vi "Teleop - Davis.vi"(10 "Match Info":T1={"Autonomous Elapsed Seconds"=0.0, "TeleOp Elapsed Seconds"=0.0, "Disabled Elapsed Seconds"=0.0, "Visited Autonomous"=FALSE, "Visited TeleOp"=FALSE, "Visited Disabled"=FALSE, "Autonomous Settings"={"Autonomous Style"=enum."Independent", "VI Refnum"=refnum}}, 11 "Call Context":T2) -> ()   [LabVIEW 2018]
doc: "This VI is called for each TeleOp packet received from the DS where the robot is not disabled. It is often used to read from the joysticks and update I/O or to update setpoints for timed control loops. It should complete and return within 20 milliseconds or it may miss DS packets."
uses:
  <vilib>/Rock Robotics/Network Tables/NT Write Numeric Array.vi
  <vilib>/Rock Robotics/Network Tables/NT Read Boolean.vi
  Robot Global Data.vi
  <vilib>/Rock Robotics/WPI/ThirdParty/Phoenix-LabVIEW/Motor Controller/Controls/CTRE_Phoenix_MotorControl_ControlMode.ctl
  <vilib>/Rock Robotics/WPI/Solenoid/WPI_SolenoidSetEnum.vi
  <vilib>/Rock Robotics/WPI/Solenoid/WPI_SolenoidValue.ctl
  <vilib>/Rock Robotics/Network Tables/NT Write Boolean.vi
  <vilib>/Rock Robotics/Network Tables/NT Write Number.vi
  <vilib>/Rock Robotics/WPI/ThirdParty/Phoenix-LabVIEW/Motor Controller/Get/CTRE_Phoenix_MotorController_GetSelectedSensorData.vi
  <vilib>/functionblocks/FB Core/FB Core.xnode
  <vilib>/functionblocks/Bistables/SR Bistable/SR Bistable.vi
  <vilib>/functionblocks/NI_FunctionBlock Libraries.lvlib
  <vilib>/Rock Robotics/Network Tables/NT Read Number.vi
  <vilib>/Rock Robotics/Network Tables/NT Write Boolean Array.vi
  <vilib>/Rock Robotics/WPI/DriverStation/WPI_DriverStationMatch Info.ctl
  <vilib>/Rock Robotics/WPI/DriverStation/WPI_DriverStationDerivedRobotMode.ctl
panel:
  in  "I Zone":dbl
  in  "F - Generally is zero for position-servo":dbl
  in  "D":dbl
  in  "I":dbl
  in  "P":dbl
  out "Sample Slider 0":dbl(slide) scale=0.0..5.0
  out "Sample Boolean 1":bool
  out "Sample Boolean 0":bool
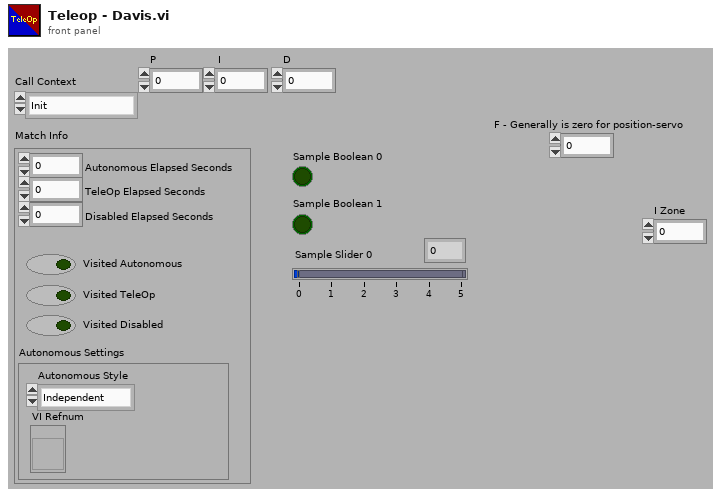
[diagram p1: front panel]
types:
  T1 = typedef "WPI_DriverStationMatch Info.ctl" = cluster{"Autonomous Elapsed Seconds":dbl, "TeleOp Elapsed Seconds":dbl, "Disabled Elapsed Seconds":dbl, "Visited Autonomous":bool, "Visited TeleOp":bool, "Visited Disabled":bool, "Autonomous Settings":cluster{"Autonomous Style":enum16{"Iterative", "Independent"}, "VI Refnum":refnum<vi>}}
  T2 = typedef "WPI_DriverStationDerivedRobotMode.ctl" = enum16{"Init", "Execute", "Stop"}
  T3 = typedef "CTRE_Phoenix_MotorControl_ControlMode.ctl" = u16
  T4 = typedef "WPI_MotorControlDeviceRef.ctl" = cluster{"DeviceStatus":errorcluster, "Type":T5, "PWM":cluster{"PWM Channel":T6, "DeadBand":T7}, "CAN":cluster{"Device Number":u8, "SetOutput VI Ref":variant, "GetOutput VI Ref":variant, "Enable VI Ref":variant, "Disable VI Ref":variant, "Data":variant}, "Invert":bool, "DIO PWM":cluster{"PWM \"Enable\" Channel":T6, "DIOChannel":T8, "PWM Rate":dbl}}
  T5 = typedef "WPI_MotorControlType.ctl" = enum16{"PWM", "CAN", "DIO PWM"}
  T6 = typedef "FPGA_DIOPWMChannel.ctl" = enum8{"PWM 0", "PWM 1", "PWM 2", "PWM 3", "PWM 4", "PWM 5", "PWM 6", "PWM 7", "PWM 8", "PWM 9", "PWM MXP 0", "PWM MXP 1", "PWM MXP 2", "PWM MXP 3", "PWM MXP 4", "PWM MXP 5", "PWM MXP 6", "PWM MXP 7", "PWM MXP 8", "PWM MXP 9", "Invalid"}
  T7 = typedef "WPI_PWMDeadband.ctl" = cluster{"Name":string, "maxPositivePwm":i32, "minPositivePwm":i32, "centerPwm":i32, "maxNegativePwm":i32, "minNegativePwm":i32, "angularRange":u16}
  T8 = typedef "FPGA_DIOChannel.ctl" = enum8{"DIO 0", "DIO 1", "DIO 2", "DIO 3", "DIO 4", "DIO 5", "DIO 6", "DIO 7", "DIO 8", "DIO 9", "DIO MXP 0", "DIO MXP 1", "DIO MXP 2", "DIO MXP 3", "DIO MXP 4", "DIO MXP 5", "DIO MXP 6", "DIO MXP 7", "DIO MXP 8", "DIO MXP 9", "DIO MXP 10", "DIO MXP 11", "DIO MXP 12", "DIO MXP 13", "DIO MXP 14", "DIO MXP 15", "SPI Port CS1", "SPI Port CS2", "SPI Port CS3", "SPI Port MISO", "SPI Port MOSI", "Invalid"}
  T9 = typedef "WPI_SwitchDevRef.ctl" = cluster{"DevStatus":errorcluster, "DIO Channel":T8, "CntIndex":T10, "Normally Closed":bool}
  T10 = typedef "FPGA_CounterCtrSystemIndex.ctl" = enum8{"Ctr 0", "Ctr 1", "Ctr 2", "Ctr 3", "Ctr 4", "Ctr 5", "Ctr 6", "Ctr 7", "Invalid"}
  T11 = typedef "WPI_SolenoidValue.ctl" = enum16{"Off", "On", "Forward", "Reverse"}
  T12 = typedef "WPI_SolenoidDevRef.ctl" = cluster{"DevStatus":errorcluster, "Pneumatics Control Module":u8, "Forward Solenoid Channel":T13, "Reverse Solenoid Channel":T13}
  T13 = typedef "WPI_SolenoidChannel.ctl" = enum8{"Solenoid 0", "Solenoid 1", "Solenoid 2", "Solenoid 3", "Solenoid 4", "Solenoid 5", "Solenoid 6", "Solenoid 7", "Invalid"}
  T14 = typedef "WPI_JoystickDevRef.ctl" = cluster{"Device":T15}
  T15 = typedef "WPI_JoystickDeviceEnum.ctl" = enum16{"USB 0", "USB 1", "USB 2", "USB 3", "USB 4", "USB 5"}
  T16 = typedef "WPI_RobotDriveDevRef.ctl" = cluster{"DevStatus":errorcluster, "Motors[]":T4[], "Square Inputs":bool, "Max Output":dbl}
  T17 = cluster{"JoystickDevRef":T14, "JoystickDevRef":T14}
  T18 = cluster{"Axes[0]":dbl, "Axes[1]":dbl, "Axes[2]":dbl, "Axes[3]":dbl, "Axes[4]":dbl, "Axes[5]":dbl, "Axes[6]":dbl, "Axes[7]":dbl, "Axes[8]":dbl}
  T19 = cluster{"Buttons[0]":bool, "Buttons[1]":bool, "Buttons[2]":bool, "Buttons[3]":bool, "Buttons[4]":bool, "Buttons[5]":bool, "Buttons[6]":bool, "Buttons[7]":bool, "Buttons[8]":bool}
  T20 = typedef "WPI_ServoDeviceRef.ctl" = cluster{"DeviceStatus":errorcluster, "PWM Channel":T6, "DeadBand":T7}
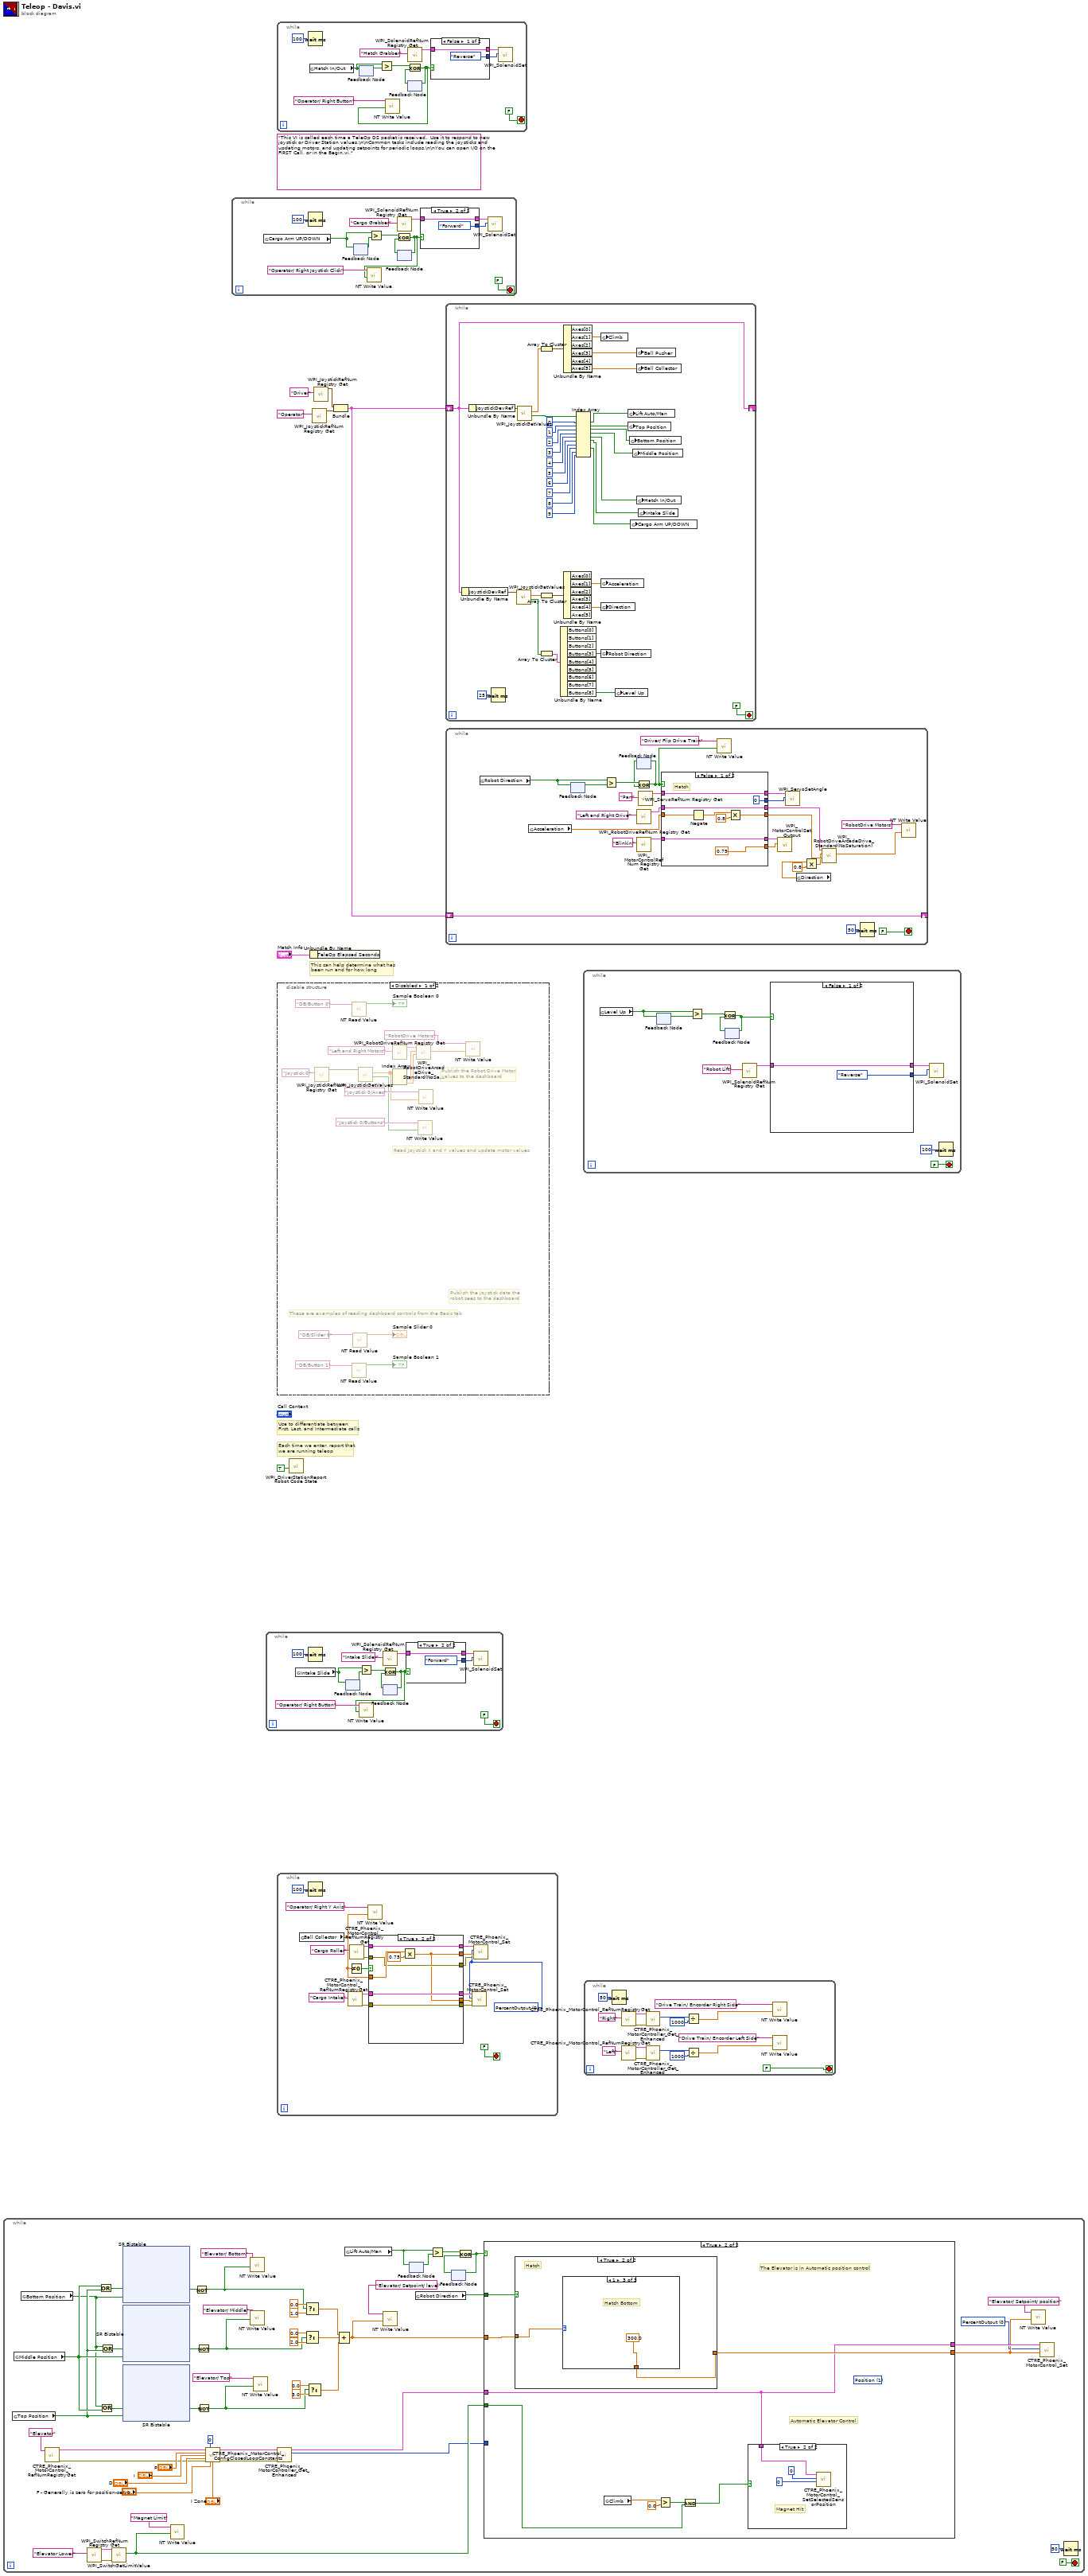
[diagram p0: block diagram]
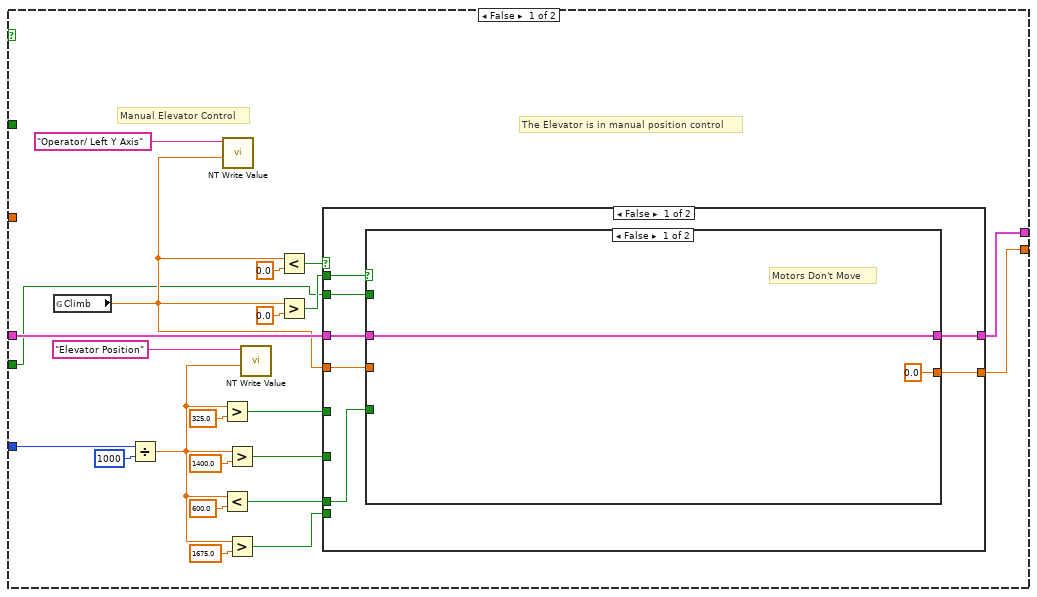
[diagram p2: hidden frame]
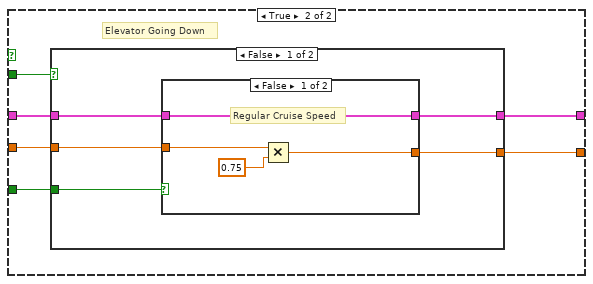
[diagram p3: hidden frame]
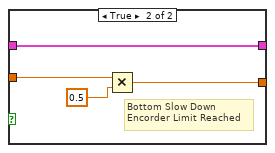
[diagram p4: hidden frame]
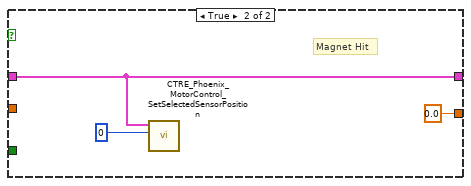
[diagram p5: hidden frame]
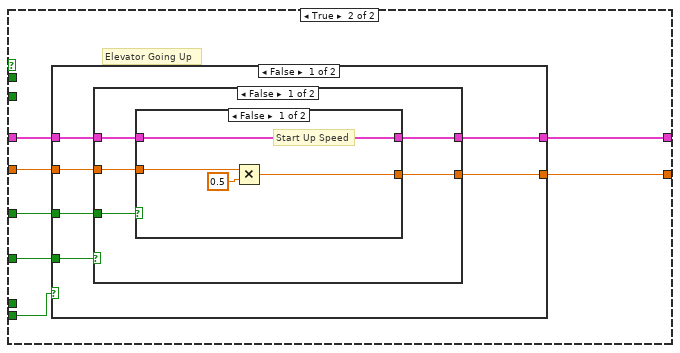
[diagram p6: hidden frame]
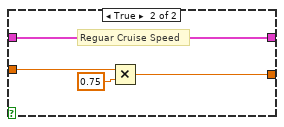
[diagram p7: hidden frame]
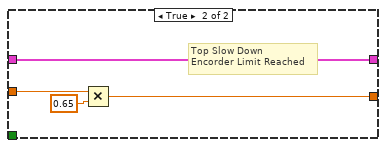
[diagram p8: hidden frame]
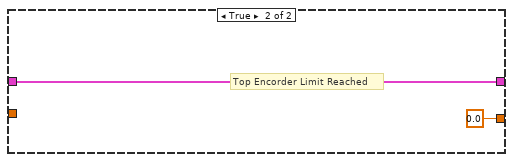
[diagram p9: hidden frame]
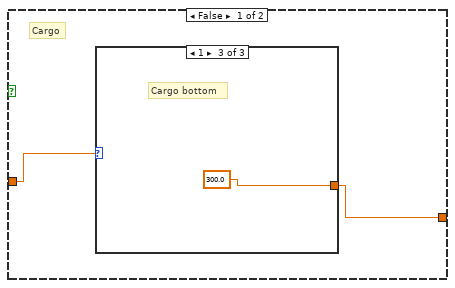
[diagram p11: hidden frame]
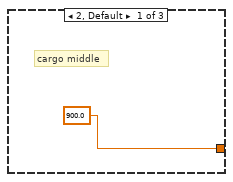
[diagram p12: hidden frame]
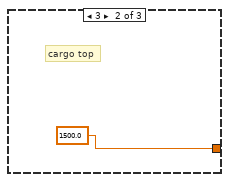
[diagram p13: hidden frame]
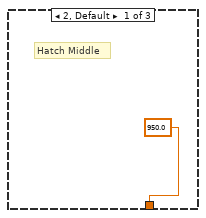
[diagram p14: hidden frame]
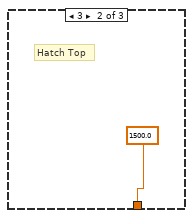
[diagram p15: hidden frame]
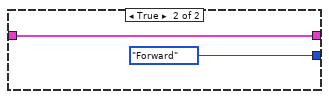
[diagram p16: hidden frame]
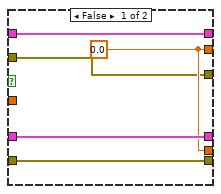
[diagram p17: hidden frame]
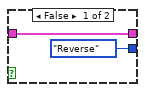
[diagram p18: hidden frame]
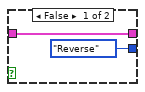
[diagram p19: hidden frame]
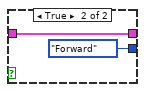
[diagram p20: hidden frame]
diagram:
  (unwired) "This VI is called each time a TeleOp DS packet is received.  Use it to respond to new joystick or Driver Station values.\n\nCommon tasks include reading the joysticks and updating motors, and updating setpoints for periodic loops.\n\nYou can open I/O on the FIRST Call, or in the Begin.vi."
  # "Each time we enter, report that\nwe are running teleop"
  # "Use to differentiate between\nFirst, Last, and Intermediate calls"
  # "This can help determine what has\nbeen run and for how long"
  n1 = while {
    stop <- FALSE stop-if-true
    w8 = T3 0 items=["PercentOutput"=0, "Position"=1, "Velocity"=2, "Current"=3, "Follower"=5, "MotionProfile"=6, "MotionMagic"=7, "MotionProfileArc"=10, "Disabled"=15] ("Control Mode")
    n2 = global read "Robot Global Data.vi" "Top Position"() -> (w12:bool)
    n3 = global read "Robot Global Data.vi" "Middle Position"() -> (w13:bool)
    n4 = global read "Robot Global Data.vi" "Bottom Position"() -> (w11:bool)
    n5 = call <vilib>:"CTRE_Phoenix_MotorControl_RefNumRegistryGet.vi"("refnum name"="Elevator") -> ("error out"=w20:errorcluster, "PhoenixMotorControlDevRef"=w31:T4)  [unwired: 9 in]
    n6 = call <vilib>:"WPI_SwitchRefNum Registry Get.vi"("refnum name"="Elevator Lower") -> ("error out"=w38:errorcluster, "SwitchDevRef"=w37:T9)  [unwired: 9 in]
    n7 = Or(x=w13, y=w12) -> (x .or. y?=w41:bool)
    n8 = Or(x=w11, y=w13) -> (x .or. y?=w39:bool)
    n9 = Or(x=w11, y=w12) -> (x .or. y?=w40:bool)
    n10 = call <vilib>:"WPI_SwitchGetLimitValue.vi"("error in (no error)"=w38, "SwitchDevRef"=w37) -> ("Switch Pressed"=w34:bool)  [unwired: 7 in, 2 out]
    n11 = xnode "SR Bistable"("reset"=w41, "set"=w11) -> ("output"=w18:bool)  [unwired: 1 in, 1 out]
    n12 = xnode "SR Bistable"("reset"=w40, "set"=w13) -> ("output"=w17:bool)  [unwired: 1 in, 1 out]
    n13 = xnode "SR Bistable"("reset"=w39, "set"=w12) -> ("output"=w16:bool)  [unwired: 1 in, 1 out]
    n14 = call-poly <vilib>:"NT Write Value.vi"("Boolean"=w34, "Name"="Magnet Limit") -> ()  [unwired: 9 in, 1 out]
    n15 = Not(x=w18) -> (.not. x?=w10:bool)
    n16 = Not(x=w17) -> (.not. x?=w14:bool)
    n17 = Not(x=w16) -> (.not. x?=w15:bool)
    n18 = call <vilib>:"CTRE_Phoenix_MotorControl_ConfigClosedLoopConstants.vi"("PhoenixMotorControlDevRef"=w31, "slotIdx"=0, "P"="P", "I"="I", "D"="D", "error in (no error)"=w20, "F"="F - Generally is zero for position-servo", "I Zone"="I Zone") -> ("PhoenixMotorControlDevRef"=w32:T4, "error out"=w19:errorcluster)  [unwired: 6 in]
    n19 = call-poly <vilib>:"NT Write Value.vi"("Boolean"=w14, "Name"="Elevator/ Middle") -> ()  [unwired: 9 in, 1 out]
    n20 = call-poly <vilib>:"NT Write Value.vi"("Boolean"=w10, "Name"="Elevator/ Bottom") -> ()  [unwired: 9 in, 1 out]
    n21 = call-poly <vilib>:"NT Write Value.vi"("Boolean"=w15, "Name"="Elevator/ Top") -> ()  [unwired: 9 in, 1 out]
    n22 = call-poly <vilib>:"CTRE_Phoenix_MotorController_Get_Enhanced.vi"("PhoenixMotorControlDevRef"=w32, "error in"=w19) -> ("PhoenixMotorControlDevRef"=w9:T4, "Position (Raw Sensor Units)"=w33:i32)  [unwired: 10 in, 2 out]
    n23 = Select(t=0.0, s=w10, f=1.0) -> (s? t:f=w53:dbl)
    n24 = Select(t=0.0, s=w14, f=2.0) -> (s? t:f=w52:dbl)
    n25 = Select(t=0.0, s=w15, f=3.0) -> (s? t:f=w51:dbl)
    n26 = Compound Arithmetic op=ADD(w53, w52, w51) -> (w23:dbl)
    n27 = global read "Robot Global Data.vi" "Lift Auto/Man"() -> (w55:bool)
    n28 = call-poly <vilib>:"NT Write Value.vi"("Numeric"=w23, "Name"="Elevator/ Setpoint/ level") -> ()  [unwired: 9 in, 1 out]
    n29 = feedback #1() -> (w57:bool)  [unwired: 1 in]
    n30 = feedback-in #1(w55) -> ()
    n31 = global read "Robot Global Data.vi" "Robot Direction"() -> (w54:bool)
    n32 = Greater?(x=w55, y=w57) -> (0:w58:bool)
    n33 = feedback #2() -> (w59:bool)  [unwired: 1 in]
    n34 = Exclusive Or(1:w59, 2:w58) -> (0:w56:bool)
    n35 = feedback-in #2(w56) -> ()
    n36 = case shown="True" w56 {
      tunnel: [w206 w276] -> w21
      tunnel: w9 -> [w205 w275]
      tunnel: [w204 w275] -> w60
      tunnel: w33 -> [w190 _]
      tunnel: w54 -> [_ w283]
      tunnel: w23 -> [_ w282]
      tunnel: w34 -> [w191 w279]
      frame False {
        # "The Elevator is in manual position control"
        # "Manual Elevator Control"
        n37 = global read "Robot Global Data.vi" "Climb"() -> (w197:dbl)
        n38 = Divide(x=w190, y=1000) -> (x/y=w196:dbl)
        n39 = Greater?(x=w196, y=325.0) -> (0:w194:bool)
        n40 = Less?(x=w196, y=600.0) -> (x < y?=w192:bool)
        n41 = call-poly <vilib>:"NT Write Value.vi"("Numeric"=w197, "Name"="Operator/ Left Y Axis") -> ()  [unwired: 9 in, 1 out]
        n42 = Greater?(x=w196, y=1400.0) -> (0:w198:bool)
        n43 = Greater?(x=w196, y=1675.0) -> (0:w199:bool)
        n44 = call-poly <vilib>:"NT Write Value.vi"("Numeric"=w196, "Name"="Elevator Position") -> ()  [unwired: 9 in, 1 out]
        n45 = Less?(x=w197, y=0.0) -> (x < y?=w200:bool)
        n46 = Greater?(x=w197, y=0.0) -> (0:w193:bool)
        n47 = case shown="False" w200 {
          tunnel: [w216 w246] -> w206
          tunnel: w205 -> [w214 w247]
          tunnel: [w215 w248] -> w204
          tunnel: w199 -> [_ w249]
          tunnel: w198 -> [_ w245]
          tunnel: w197 -> [w212 w244]
          tunnel: w194 -> [_ w243]
          tunnel: w193 -> [w218 _]
          tunnel: w191 -> [w217 _]
          tunnel: w192 -> [w213 _]
          frame False {
            n48 = case shown="False" w218 {
              tunnel: w217 -> [_ w226]
              tunnel: [0.0 ("Climb") w225] -> w216
              tunnel: [w220 w224] -> w215
              tunnel: w214 -> [w220 w223]
              tunnel: w213 -> [_ w222]
              tunnel: w212 -> [_ w221]
              frame False {
                # "Motors Don't Move"
              }
              frame True {
                # "Elevator Going Down"
                n49 = case shown="False" w226 {
                  tunnel: [w230 0.0 ("Climb")] -> w225
                  tunnel: [w228 w240] -> w224
                  tunnel: w223 -> [w227 w240]
                  tunnel: w222 -> [w231 _]
                  tunnel: w221 -> [w229 _]
                  frame False {
                    n50 = case shown="False" w231 {
                      tunnel: [w235 w239] -> w230
                      tunnel: w229 -> [w234 w238]
                      tunnel: [w233 w236] -> w228
                      tunnel: w227 -> [w233 w236]
                      frame False {
                        # "Regular Cruise Speed"
                        n51 = Multiply(x=w234, y=0.75) -> (x*y=w235:dbl)
                      }
                      frame True {
                        # "Bottom Slow Down\nEncorder Limit Reached"
                        n52 = Multiply(x=w238, y=0.5) -> (x*y=w239:dbl)
                      }
                    }
                  }
                  frame True {
                    # "Magnet Hit"
                    n53 = call <vilib>:"CTRE_Phoenix_MotorControl_SetSelectedSensorPosition.vi"("New Sensor Position"=0, "PhoenixMotorControlDevRef"=w240) -> ()  [unwired: 8 in, 2 out]
                  }
                }
              }
            }
          }
          frame True {
            # "Elevator Going Up"
            n54 = case shown="False" w249 {
              tunnel: [w254 w274] -> w248
              tunnel: w247 -> [w253 w274]
              tunnel: [w252 0.0 ("Climb")] -> w246
              tunnel: w245 -> [w255 _]
              tunnel: w244 -> [w251 _]
              tunnel: w243 -> [w250 _]
              frame False {
                n55 = case shown="False" w255 {
                  tunnel: [w257 w272] -> w254
                  tunnel: w253 -> [w256 w272]
                  tunnel: [w259 w271] -> w252
                  tunnel: w251 -> [w258 w270]
                  tunnel: w250 -> [w260 _]
                  frame False {
                    n56 = case shown="False" w260 {
                      tunnel: [w264 w268] -> w259
                      tunnel: w258 -> [w263 w267]
                      tunnel: [w261 w266] -> w257
                      tunnel: w256 -> [w261 w266]
                      frame False {
                        # "Start Up Speed"
                        n57 = Multiply(x=w263, y=0.5) -> (x*y=w264:dbl)
                      }
                      frame True {
                        # "Reguar Cruise Speed"
                        n58 = Multiply(x=w267, y=0.75) -> (x*y=w268:dbl)
                      }
                    }
                  }
                  frame True {
                    # "Top Slow Down\nEncorder Limit Reached"
                    n59 = Multiply(x=w270, y=0.65) -> (x*y=w271:dbl)
                  }
                }
              }
              frame True {
                # "Top Encorder Limit Reached"
              }
            }
          }
        }
      }
      frame True {
        (unwired) T3 1 items=["PercentOutput"=0, "Position"=1, "Velocity"=2, "Current"=3, "Follower"=5, "MotionProfile"=6, "MotionMagic"=7, "MotionProfileArc"=10, "Disabled"=15] ("Control Mode")
        # "The Elevator is in Automatic position control"
        # "Automatic Elevator Control"
        n60 = case shown="True" w283 {
          tunnel: w282 -> [w288 w293]
          tunnel: [w287 w292] -> w276
          frame False {
            # "Cargo"
            n61 = case shown="1" w288 {
              tunnel: [900.0 ("setpoint") 1500.0 ("setpoint") 300.0 ("setpoint")] -> w287
              frame 2, Default {
                # "cargo middle"
              }
              frame 3 {
                # "cargo top"
              }
              frame 1 {
                # "Cargo bottom"
              }
            }
          }
          frame True {
            # "Hatch"
            n62 = case shown="1" w293 {
              tunnel: [950.0 ("setpoint") 1500.0 ("setpoint") 300.0 ("setpoint")] -> w292
              frame 2, Default {
                # "Hatch Middle"
              }
              frame 3 {
                # "Hatch Top"
              }
              frame 1 {
                # "Hatch Bottom"
              }
            }
          }
        }
        n63 = global read "Robot Global Data.vi" "Climb"() -> (w280:dbl)
        n64 = Greater?(x=w280, y=0.0) -> (0:w278:bool)
        n65 = And(x=w278, y=w279) -> (x .and. y?=w277:bool)
        n66 = case shown="True" w277 {
          tunnel: w275 -> [_ w286]
          frame False {
          }
          frame True {
            # "Magnet Hit"
            n67 = call <vilib>:"CTRE_Phoenix_MotorControl_SetSelectedSensorPosition.vi"("pidLoopIdx"=u32 0, "New Sensor Position"=0, "PhoenixMotorControlDevRef"=w286) -> ()  [unwired: 7 in, 2 out]
          }
        }
      }
    }
    n68 = call-poly <vilib>:"NT Write Value.vi"("Numeric"=w21, "Name"="Elevator/ Setpoint/ position") -> ()  [unwired: 9 in, 1 out]
    n69 = call <vilib>:"CTRE_Phoenix_MotorControl_Set.vi"("Output"=w21, "Control Mode"=w8, "PhoenixMotorControlDevRef"=w60) -> ()  [unwired: 7 in, 2 out]
    n70 = Wait (ms)(milliseconds to wait=u32 50) -> ()  [unwired: 1 out]
  }
  n71 = while {
    stop <- FALSE stop-if-true
    n72 = global read "Robot Global Data.vi" "Cargo Arm UP/DOWN"() -> (w298:bool)
    n73 = Wait (ms)(milliseconds to wait=u32 100) -> ()  [unwired: 1 out]
    n74 = feedback #3() -> (w302:bool)  [unwired: 1 in]
    n75 = feedback-in #3(w298) -> ()
    n76 = Greater?(x=w298, y=w302) -> (0:w303:bool)
    n77 = call <vilib>:"WPI_SolenoidRefNum Registry Get.vi"("refnum name"="Cargo Grabber") -> ("SolenoidDevRef"=w306:T12)  [unwired: 9 in, 1 out]
    n78 = feedback #4() -> (w304:bool)  [unwired: 1 in]
    n79 = Exclusive Or(1:w304, 2:w303) -> (0:w297:bool)
    n80 = call-poly <vilib>:"NT Write Value.vi"("Boolean"=w297, "Name"="Operator/ Right Joystick Click") -> ()  [unwired: 9 in, 1 out]
    n81 = feedback-in #4(w297) -> ()
    n82 = case shown="True" w297 {
      tunnel: w306 -> [w310 w312]
      tunnel: [w310 w312] -> w307
      tunnel: [WPI_SolenoidValue."Reverse" ("Value") WPI_SolenoidValue."Forward" ("Value")] -> w308
      frame False {
      }
      frame True {
      }
    }
    n83 = call-poly <vilib>:"WPI_SolenoidSet.vi"("Value"=w308, "SolenoidDevRef"=w307) -> ()  [unwired: 8 in, 2 out]
  }
  n84 = while {
    stop <- FALSE stop-if-true
    n85 = global read "Robot Global Data.vi" "Intake Slide"() -> (w317:bool)
    n86 = Wait (ms)(milliseconds to wait=u32 100) -> ()  [unwired: 1 out]
    n87 = feedback #5() -> (w324:bool)  [unwired: 1 in]
    n88 = feedback-in #5(w317) -> ()
    n89 = Greater?(x=w317, y=w324) -> (0:w323:bool)
    n90 = call <vilib>:"WPI_SolenoidRefNum Registry Get.vi"("refnum name"="Intake Slider") -> ("SolenoidDevRef"=w320:T12)  [unwired: 9 in, 1 out]
    n91 = feedback #6() -> (w322:bool)  [unwired: 1 in]
    n92 = Exclusive Or(1:w322, 2:w323) -> (0:w313:bool)
    n93 = call-poly <vilib>:"NT Write Value.vi"("Boolean"=w313, "Name"="Operator/ Right Button") -> ()  [unwired: 9 in, 1 out]
    n94 = feedback-in #6(w313) -> ()
    n95 = case shown="True" w313 {
      tunnel: w320 -> [w326 w328]
      tunnel: [w326 w328] -> w319
      tunnel: [WPI_SolenoidValue."Reverse" ("Value") WPI_SolenoidValue."Forward" ("Value")] -> w318
      frame False {
      }
      frame True {
      }
    }
    n96 = call-poly <vilib>:"WPI_SolenoidSet.vi"("Value"=w318, "SolenoidDevRef"=w319) -> ()  [unwired: 8 in, 2 out]
  }
  n97 = while {
    stop <- FALSE stop-if-true
    n98 = Wait (ms)(milliseconds to wait=u32 100) -> ()  [unwired: 1 out]
    n99 = global read "Robot Global Data.vi" "Hatch In/Out"() -> (w330:bool)
    n100 = feedback #7() -> (w333:bool)  [unwired: 1 in]
    n101 = feedback-in #7(w330) -> ()
    n102 = Greater?(x=w330, y=w333) -> (0:w332:bool)
    n103 = call <vilib>:"WPI_SolenoidRefNum Registry Get.vi"("refnum name"="Hatch Grabber") -> ("SolenoidDevRef"=w339:T12)  [unwired: 9 in, 1 out]
    n104 = feedback #8() -> (w331:bool)  [unwired: 1 in]
    n105 = Exclusive Or(1:w331, 2:w332) -> (0:w329:bool)
    n106 = call-poly <vilib>:"NT Write Value.vi"("Boolean"=w329, "Name"="Operator/ Right Button") -> ()  [unwired: 9 in, 1 out]
    n107 = feedback-in #8(w329) -> ()
    n108 = case shown="False" w329 {
      tunnel: w339 -> [w342 w344]
      tunnel: [w342 w344] -> w338
      tunnel: [WPI_SolenoidValue."Reverse" ("Value") WPI_SolenoidValue."Forward" ("Value")] -> w337
      frame False {
      }
      frame True {
      }
    }
    n109 = call-poly <vilib>:"WPI_SolenoidSet.vi"("Value"=w337, "SolenoidDevRef"=w338) -> ()  [unwired: 8 in, 2 out]
  }
  n110 = disable-structure shown="Disabled" {
    frame Disabled {
      # "These are examples of reading dashboard controls from the Basic tab"
      # "Publish the Robot Drive Motor\nvalues to the dashboard"
      # "Publish the joystick data the\nrobot sees to the dashboard"
      # "Read Joystick X and Y values and update motor values"
      n111 = call <vilib>:"WPI_JoystickRefNum Registry Get.vi"("refnum name"="Joystick 0") -> ("JoystickDevRef"=w358:T14)  [unwired: 1 in, 9 out]
      n112 = call-poly <vilib>:"NT Read Value.vi"("Name"="DB/Button 0" ("refnum name")) -> ("Boolean"=→"Sample Boolean 0":bool)  [unwired: 9 in, 1 out]
      n113 = call-poly <vilib>:"NT Read Value.vi"("Name"="DB/Button 1" ("refnum name")) -> ("Boolean"=→"Sample Boolean 1":bool)  [unwired: 9 in, 1 out]
      n114 = call-poly <vilib>:"NT Read Value.vi"("Name"="DB/Slider 0" ("refnum name")) -> ("Numeric"=→"Sample Slider 0":dbl)  [unwired: 9 in, 1 out]
      n115 = call <vilib>:"WPI_JoystickGetValues.vi"("JoystickDevRef"=w358) -> ("Buttons"=w353:bool[], "Axes"=w354:dbl[])  [unwired: 6 in, 3 out]
      n116 = call <vilib>:"WPI_RobotDriveRefNum Registry Get.vi"("refnum name"="Left and Right Motors") -> ("RobotDriveDevRef"=w361:T16)  [unwired: 1 in, 9 out]
      n117 = Index Array(array=w354) -> (element #1=w360:dbl, element #2=w357:dbl)  [unwired: 2 in]
      n118 = call <vilib>:"WPI_RobotDriveArcadeDrive_Standard(NoSaturation).vi"("Y axis value"=w357, "X axis value"=w360, "RobotDriveDevRef"=w361) -> ("Motor Values"=w346:dbl[])  [unwired: 1 in, 7 out]
      n119 = call-poly <vilib>:"NT Write Value.vi"("Boolean Array"=w353, "Name"="Joystick 0/Buttons") -> ()  [unwired: 9 in, 1 out]
      n120 = call-poly <vilib>:"NT Write Value.vi"("Numeric Array"=w354, "Name"="Joystick 0/Axes") -> ()  [unwired: 9 in, 1 out]
      n121 = call-poly <vilib>:"NT Write Value.vi"("Numeric Array"=w346, "Name"="RobotDrive Motors") -> ()  [unwired: 9 in, 1 out]
    }
    frame Enabled {
    }
  }
  n122 = while {
    stop <- FALSE stop-if-true
    w368 = T3 0 items=["PercentOutput"=0, "Position"=1, "Velocity"=2, "Current"=3, "Follower"=5, "MotionProfile"=6, "MotionMagic"=7, "MotionProfileArc"=10, "Disabled"=15] ("Control Mode")
    n123 = global read "Robot Global Data.vi" "Ball Collector"() -> (w373:dbl)
    n124 = Wait (ms)(milliseconds to wait=u32 100) -> ()  [unwired: 1 out]
    n125 = call <vilib>:"CTRE_Phoenix_MotorControl_RefNumRegistryGet.vi"("refnum name"="Cargo Intake") -> ("error out"=w364:errorcluster, "PhoenixMotorControlDevRef"=w369:T4)  [unwired: 9 in]
    n126 = Not Equal To 0?(x=w373) -> (x != 0?=w380:bool)
    n127 = call <vilib>:"CTRE_Phoenix_MotorControl_RefNumRegistryGet.vi"("refnum name"="Cargo Roller") -> ("error out"=w366:errorcluster, "PhoenixMotorControlDevRef"=w377:T4)  [unwired: 9 in]
    n128 = call-poly <vilib>:"NT Write Value.vi"("Numeric"=w373, "Name"="Operator/ Right Y Axis") -> ()  [unwired: 9 in, 1 out]
    n129 = case shown="True" w380 {
      tunnel: w377 -> [w385 w392]
      tunnel: [w385 w392] -> w378
      tunnel: w373 -> [_ w391]
      tunnel: [w383 w386] -> w379
      tunnel: [w384 w389] -> w370
      tunnel: w369 -> [w384 w389]
      tunnel: [w381 w388] -> w367
      tunnel: w366 -> [w381 w388]
      tunnel: [w382 w387] -> w365
      tunnel: w364 -> [w382 w387]
      tunnel: [w383 w386] -> w363
      frame False {
        w383 = 0.0 ("Climb")
      }
      frame True {
        n130 = Multiply(x=w391, y=0.75) -> (x*y=w386:dbl)
      }
    }
    n131 = call <vilib>:"CTRE_Phoenix_MotorControl_Set.vi"("error in (no error)"=w365, "Output"=w363, "Control Mode"=w368, "PhoenixMotorControlDevRef"=w370) -> ()  [unwired: 6 in, 2 out]
    n132 = call <vilib>:"CTRE_Phoenix_MotorControl_Set.vi"("error in (no error)"=w367, "Output"=w379, "Control Mode"=w368, "PhoenixMotorControlDevRef"=w378) -> ()  [unwired: 6 in, 2 out]
  }
  n133 = call <vilib>:"WPI_DriverStationReport Robot Code State.vi"("TeleOp"=TRUE ("Autonomous")) -> ()  [unwired: 10 in, 1 out]
  n134 = Unbundle By Name("Match Info") -> ()  [unwired: 1 out]
  n135 = call <vilib>:"WPI_JoystickRefNum Registry Get.vi"("refnum name"="Operator") -> ("JoystickDevRef"=w3:T14)  [unwired: 1 in, 9 out]
  n136 = call <vilib>:"WPI_JoystickRefNum Registry Get.vi"("refnum name"="Driver") -> ("JoystickDevRef"=w4:T14)  [unwired: 1 in, 9 out]
  n137 = Bundle("JoystickDevRef"=w4, "JoystickDevRef"=w3) -> (w2:T17)  [unwired: 1 out]
  n138 = while {
    shift-right: [w420] -> _
    shift-left: w2 -> [w420]
    stop <- FALSE stop-if-true
    n139 = Unbundle By Name(w420) -> ("JoystickDevRef"=w426:T14)
    n140 = Unbundle By Name(w420) -> ("JoystickDevRef"=w417:T14)
    n141 = Wait (ms)(milliseconds to wait=u32 25) -> ()  [unwired: 1 out]
    n142 = call <vilib>:"WPI_JoystickGetValues.vi"("JoystickDevRef"=w426) -> ("Buttons"=w423:bool[], "Axes"=w425:dbl[])  [unwired: 6 in, 3 out]
    n143 = call <vilib>:"WPI_JoystickGetValues.vi"("JoystickDevRef"=w417) -> ("Buttons"=w411:bool[], "Axes"=w416:dbl[])  [unwired: 6 in, 3 out]
    n144 = Array To Cluster(array=w416) -> (cluster=w415:T18)
    n145 = Array To Cluster(array=w425) -> (cluster=w424:T18)
    n146 = Array To Cluster(array=w423) -> (cluster=w422:T19)
    n147 = Unbundle By Name(w422) -> ("Buttons[3]"=w419:bool, "Buttons[8]"=w393:bool)  [unwired: 7 out]
    n148 = Unbundle By Name(w424) -> ("Axes[1]"=w421:dbl, "Axes[4]"=w418:dbl)  [unwired: 4 out]
    n149 = Unbundle By Name(w415) -> ("Axes[1]"=w414:dbl, "Axes[3]"=w412:dbl, "Axes[5]"=w413:dbl)  [unwired: 3 out]
    n150 = Index Array(array=w411, index #1=0 ("index"), index #2=1 ("index"), index #3=2 ("index"), index #4=3 ("index"), index #5=4 ("index"), index #6=5 ("index"), index #7=6 ("index"), index #8=7 ("index"), index #9=8 ("index"), index #10=9 ("index")) -> (element #1=w400:bool, element #2=w399:bool, element #3=w398:bool, element #4=w397:bool, element #5=w396:bool, element #6=w395:bool, element #8=w394:bool)  [unwired: 3 out]
    n151 = global write "Robot Global Data.vi" "Climb"(w414) -> ()
    n152 = global write "Robot Global Data.vi" "Acceleration"(w421) -> ()
    n153 = global write "Robot Global Data.vi" "Direction"(w418) -> ()
    n154 = global write "Robot Global Data.vi" "Robot Direction"(w419) -> ()
    n155 = global write "Robot Global Data.vi" "Level Up"(w393) -> ()
    n156 = global write "Robot Global Data.vi" "Lift Auto/Man"(w400) -> ()
    n157 = global write "Robot Global Data.vi" "Top Position"(w399) -> ()
    n158 = global write "Robot Global Data.vi" "Bottom Position"(w398) -> ()
    n159 = global write "Robot Global Data.vi" "Cargo Arm UP/DOWN"(w394) -> ()
    n160 = global write "Robot Global Data.vi" "Middle Position"(w397) -> ()
    n161 = global write "Robot Global Data.vi" "Ball Pusher"(w412) -> ()
    n162 = global write "Robot Global Data.vi" "Ball Collector"(w413) -> ()
    n163 = global write "Robot Global Data.vi" "Hatch In/Out"(w396) -> ()
    n164 = global write "Robot Global Data.vi" "Intake Slide"(w395) -> ()
  }
  n165 = while {
    shift-right: [w448] -> _
    shift-left: w2 -> [w448]
    stop <- FALSE stop-if-true
    n166 = global read "Robot Global Data.vi" "Robot Direction"() -> (w453:bool)
    n167 = global read "Robot Global Data.vi" "Acceleration"() -> (w450:dbl)
    n168 = feedback #9() -> (w454:bool)  [unwired: 1 in]
    n169 = feedback-in #9(w453) -> ()
    n170 = Greater?(x=w453, y=w454) -> (0:w452:bool)
    n171 = feedback #10() -> (w451:bool)  [unwired: 1 in]
    n172 = Exclusive Or(1:w451, 2:w452) -> (0:w434:bool)
    n173 = feedback-in #10(w434) -> ()
    n174 = call <vilib>:"WPI_RobotDriveRefNum Registry Get.vi"("refnum name"="Left and Right Drive") -> ("RobotDriveDevRef"=w440:T16)  [unwired: 9 in, 1 out]
    n175 = call <vilib>:"WPI_MotorControlRefNum Registry Get.vi"("refnum name"="Blinkin") -> ("MotorControlDevRef"=w431:T4)  [unwired: 9 in, 1 out]
    n176 = call <vilib>:"WPI_ServoRefNum Registry Get.vi"("refnum name"="Pan") -> ("ServoDeviceRef"=w446:T20)  [unwired: 9 in, 1 out]
    n177 = case shown="False" w434 {
      tunnel: w450 -> [w464 w468]
      tunnel: [w460 w469] -> w438
      tunnel: w446 -> [w463 w472]
      tunnel: [w463 w472] -> w445
      tunnel: [0 ("Angle") 180 ("Angle")] -> w444
      tunnel: w440 -> [w461 w470]
      tunnel: [w461 w470] -> w439
      tunnel: w431 -> [w457 w466]
      tunnel: [w457 w466] -> w430
      tunnel: [0.79 ("Output") 0.63 ("Output")] -> w429
      frame False {
        # "Hatch"
        n178 = Negate(x=w464) -> (-x=w459:dbl)
        n179 = Multiply(x=w459, y=0.8) -> (x*y=w460:dbl)
      }
      frame True {
        # "Cargo"
        n180 = Multiply(x=w468, y=0.9) -> (x*y=w469:dbl)
      }
    }
    n181 = call-poly <vilib>:"NT Write Value.vi"("Boolean"=w434, "Name"="Driver/ Flip Drive Train") -> ()  [unwired: 9 in, 1 out]
    n182 = call <vilib>:"WPI_MotorControlSetOutput.vi"("Output"=w429, "MotorControlDevRef"=w430) -> ()  [unwired: 7 in, 3 out]
    n183 = call <vilib>:"WPI_ServoSetAngle.vi"("Angle"=w444, "ServoDeviceRef"=w445) -> ()  [unwired: 8 in, 2 out]
    n184 = global read "Robot Global Data.vi" "Direction"() -> (w435:dbl)
    n185 = Multiply(x=w435, y=0.8) -> (x*y=w436:dbl)
    n186 = call <vilib>:"WPI_RobotDriveArcadeDrive_Standard(NoSaturation).vi"("Y axis value"=w438, "X axis value"=w436, "RobotDriveDevRef"=w439) -> ("Motor Values"=w443:dbl[])  [unwired: 1 in, 7 out]
    n187 = Wait (ms)(milliseconds to wait=u32 50) -> ()  [unwired: 1 out]
    n188 = call-poly <vilib>:"NT Write Value.vi"("Numeric Array"=w443, "Name"="RobotDrive Motors") -> ()  [unwired: 9 in, 1 out]
  }
  n189 = while {
    stop <- FALSE stop-if-true
    n190 = global read "Robot Global Data.vi" "Level Up"() -> (w478:bool)
    n191 = feedback #11() -> (w481:bool)  [unwired: 1 in]
    n192 = feedback-in #11(w478) -> ()
    n193 = Greater?(x=w478, y=w481) -> (0:w480:bool)
    n194 = feedback #12() -> (w479:bool)  [unwired: 1 in]
    n195 = Exclusive Or(1:w479, 2:w480) -> (0:w477:bool)
    n196 = feedback-in #12(w477) -> ()
    n197 = call <vilib>:"WPI_SolenoidRefNum Registry Get.vi"("refnum name"="Robot Lift") -> ("SolenoidDevRef"=w475:T12)  [unwired: 9 in, 1 out]
    n198 = case shown="False" w477 {
      tunnel: w475 -> [w485 w487]
      tunnel: [w485 w487] -> w474
      tunnel: [WPI_SolenoidValue."Reverse" ("Value") WPI_SolenoidValue."Forward" ("Value")] -> w473
      frame False {
      }
      frame True {
      }
    }
    n199 = call-poly <vilib>:"WPI_SolenoidSet.vi"("Value"=w473, "SolenoidDevRef"=w474) -> ()  [unwired: 8 in, 2 out]
    n200 = Wait (ms)(milliseconds to wait=u32 100) -> ()  [unwired: 1 out]
  }
  n201 = while {
    stop <- FALSE stop-if-true
    n202 = Wait (ms)(milliseconds to wait=u32 50) -> ()  [unwired: 1 out]
    n203 = call <vilib>:"CTRE_Phoenix_MotorControl_RefNumRegistryGet.vi"("refnum name"="Right") -> ("error out"=w492:errorcluster, "PhoenixMotorControlDevRef"=w491:T4)  [unwired: 9 in]
    n204 = call <vilib>:"CTRE_Phoenix_MotorControl_RefNumRegistryGet.vi"("refnum name"="Left") -> ("error out"=w501:errorcluster, "PhoenixMotorControlDevRef"=w502:T4)  [unwired: 9 in]
    n205 = call-poly <vilib>:"CTRE_Phoenix_MotorController_Get_Enhanced.vi"("PhoenixMotorControlDevRef"=w491, "error in"=w492) -> ("Position (Raw Sensor Units)"=w493:i32)  [unwired: 10 in, 3 out]
    n206 = call-poly <vilib>:"CTRE_Phoenix_MotorController_Get_Enhanced.vi"("PhoenixMotorControlDevRef"=w502, "error in"=w501) -> ("Position (Raw Sensor Units)"=w500:i32)  [unwired: 10 in, 3 out]
    n207 = Divide(x=w493, y=1000) -> (x/y=w495:dbl)
    n208 = Divide(x=w500, y=1000) -> (x/y=w498:dbl)
    n209 = call-poly <vilib>:"NT Write Value.vi"("Numeric"=w495, "Name"="Drive Train/ Encorder Right Side") -> ()  [unwired: 9 in, 1 out]
    n210 = call-poly <vilib>:"NT Write Value.vi"("Numeric"=w498, "Name"="Drive Train/ Encorder Left Side") -> ()  [unwired: 9 in, 1 out]
  }
